vi "Pop.vi"(11 "Command Text":string) -> (2 "Command Info":string, 3 "Command Type":string)   [LabVIEW 2019, in "PathCommands.lvclass"]
uses:
  PathCommands.lvclass
  <vilib>/Utility/error.llb/whitespace.ctl
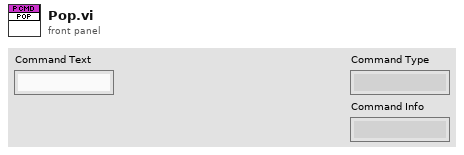
[diagram p1: front panel]
types:
  T1 = typedef "whitespace.ctl" = u16
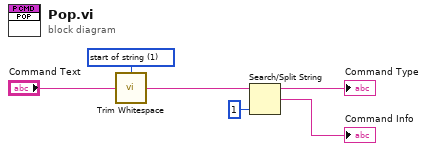
[diagram p0: block diagram]
diagram:
  w6 = T1 1 items=["both", "start of string", "end of string"] ("location (both)")
  n1 = call <vilib>:"Trim Whitespace.vi"("string"="Command Text", "location (both)"=w6) -> ("trimmed string"=w4:string)
  n2 = Search/Split String(string=w4, offset (0)=1) -> (substring before match=→"Command Type":string, match + rest of string=→"Command Info":string)  [unwired: 1 in, 1 out]
